vi "COMI Set Counter.vi"(5 "load_value":u16, 6 "bcd_bin":i32, 7 "op":i32, 9 "rw":i32, 10 "ch":i32, 11 "hDevice":u32) -> (3 "hDevice out":u32)   [LabVIEW 2017, in "Comidll.lvlib"]
doc: "void (COMI_SetCounter) (HANDLE hDevice, int ch, int rw, int op, int bcd_bin, unsigned short load_value);"
uses:
  <userlib>/Comidll/Comidll.lvlib
  <userlib>/Comidll/Comidll.dll
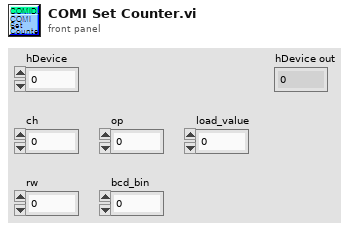
[diagram p1: front panel]
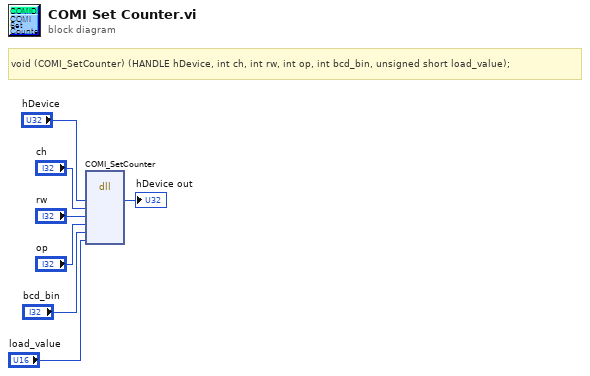
[diagram p0: block diagram]
diagram:
  # "void\t(COMI_SetCounter) (HANDLE hDevice, int ch, int rw, int op, int bcd_bin, unsigned short load_value);"
  n1 = dll-call lib="C:/Program Files/National Instruments/LabVIEW 2017/user.lib/Comidll/Comidll.*" fn="COMI_SetCounter"("hDevice"="hDevice", "ch"="ch", "rw"="rw", "op"="op", "bcd_bin"="bcd_bin", "load_value"="load_value") -> ("hDevice"=→"hDevice out":u32)  [unwired: 9 in, 2 out]
